vi "ESR Scanner - pulsed optimizer.vi"(0 "ESR Parameters":T1={"Window 1 time (s)"=0.012, "Window 2 time (s)"=5e-06, "Window 3 time (s) "=0.02, "Window 4 time (s)"=5e-07, "Window 4 channels"=[TRUE, FALSE, FALSE, TRUE], "Window 3 channels"=[TRUE, FALSE, TRUE, TRUE], "Window 2 channels"=[TRUE, FALSE, FALSE, TRUE], "Window 1 channels"=[TRUE, TRUE, FALSE, TRUE], "Path to ESR Burner"=path "C:/Users/Loncar/Desktop/ESR VIs - Srujan/Sam Kim/PB/ESRFreq.exe"}, 1 "MW start freq (GHz)":dbl=2.84, 2 "MW stop freq (GHz)":dbl=2.9, 3 "# freq points":i32=61, 4 "# scans before track":i32=50, 5 "#scan iterations":i32=50, 6 "IntGraph Refnum":refnum<vi>, 7 "Optimize Parameters":T2={"Volt Step"={"X"=0.01, "Y"=0.01, "Z"=0.0}, "Num Iterations"=1, "Dwell Time (ms)"=100, "Volts Range"={"X"=0.1, "Y"=0.1, "Z"=0.0}, "Method"={"X"=enum."Max", "Y"=enum."Max"}} {"Volts Range"."Z" min=0.0; "Volts Range"."Y" min=0.0; "Volts Range"."X" min=0.0; "Dwell Time (ms)" min=0; "Num Iterations" min=1 step=1; "Volt Step"."Z" min=0.0; "Volt Step"."Y" min=1e-06; "Volt Step"."X" min=1e-06}, 8 "XY Graph Refnum":refnum<vi>, 14 "Save avg spectrum data to spreadsheet?":bool, 15 "Path for avg spectrum spreadsheet":path=path "C:/experiment/data/may_15_2012/SIL1_NV1_pippin_uW_off", 16 "Save avg spectrum graph?":bool, 17 "Path for avg spectrum graph":path=path "C:/experiment/data/may_15_2012/SIL1_NV1_pippin_uW_off") -> ()   [LabVIEW 2012]
uses:
  Strict Type Def - Optimize Parameters Cluster.ctl
  ESR Window Parameters.ctl
  <vilib>/DAQmx/read.llb/DAQmx Read (Counter 1D U32 1Chan NSamp).vi
  Channels.vi
  <vilib>/DAQmx/miscellaneous.llb/DAQmx Fill In Error Info.vi
  Global Vars.vi
  <vilib>/Analysis/baseanly.llb/Mean (DBL).vi
  <vilib>/Utility/file.llb/Write To Spreadsheet File (DBL).vi
  <vilib>/Analysis/NI_AALBase.lvlib
panel:
  out "Counts vs. frequency":i32[][](graph)
  out "Avg ESR spectrum":cluster{"Y":dbl[], "Y":dbl[]}[](graph)
  # "Note:\nThis is not a standalone program. It is called from ScannerUI"
  # "Default PB connections:\nPB0 - MW switch\nPB1 - MW freq step\nPB2 - Counter sample clk\nPB3 - Green AOM"
  # "VI for ESR spectrum measurement\n08/26/2013, Srujan Meesala\n12/18/2013, Samuel Kim"
  # "Stop experiment and\nreset PulseBlaster"
  # "MW freq step\ndwell time"
  # "MW freq step"
  # "Wait"
  # "Fluorescence\ncounting"
  # "Ctr sample clk"
  # "Wait"
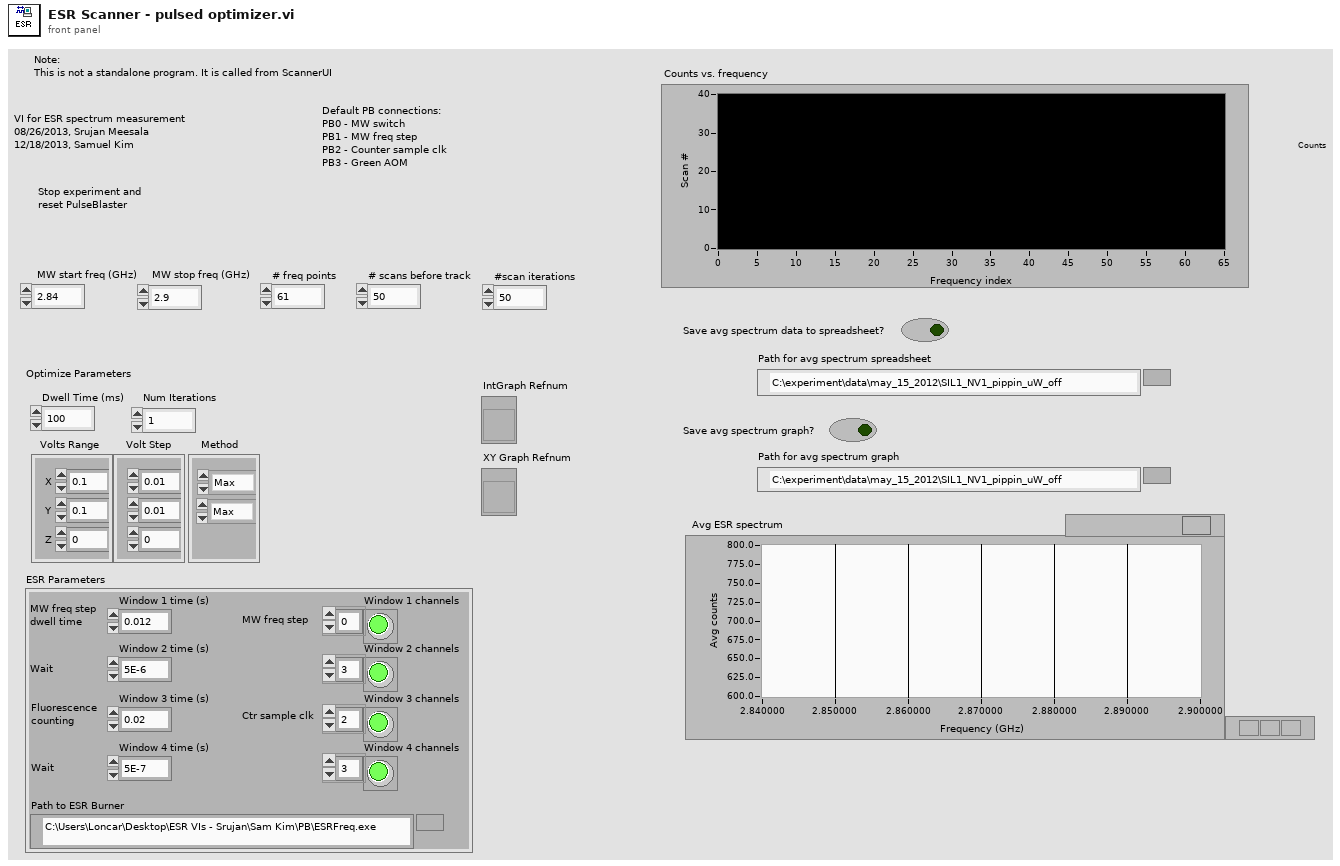
[diagram p1: front panel]
types:
  T1 = typedef "ESR Window Parameters.ctl" = cluster{"Window 1 time (s)":dbl, "Window 2 time (s)":dbl, "Window 3 time (s) ":dbl, "Window 4 time (s)":dbl, "Window 4 channels":bool[], "Window 3 channels":bool[], "Window 2 channels":bool[], "Window 1 channels":bool[], "Path to ESR Burner":path}
  T2 = typedef "Strict Type Def - Optimize Parameters Cluster.ctl" = cluster{"Volt Step":cluster{"X":dbl, "Y":dbl, "Z":dbl}, "Num Iterations":i32, "Dwell Time (ms)":i32, "Volts Range":cluster{"X":dbl, "Y":dbl, "Z":dbl}, "Method":cluster{"X":enum16{"Max", "Gaussian"}, "Y":enum16{"Max", "Gaussian"}}}
  T3 = typedef "imagedata.ctl" = cluster{"image type":i32, "image depth":i32, "image":u8[], "mask":u8[], "colors":u32[], "Rectangle":cluster{"left":i16, "top":i16, "right":i16, "bottom":i16}}
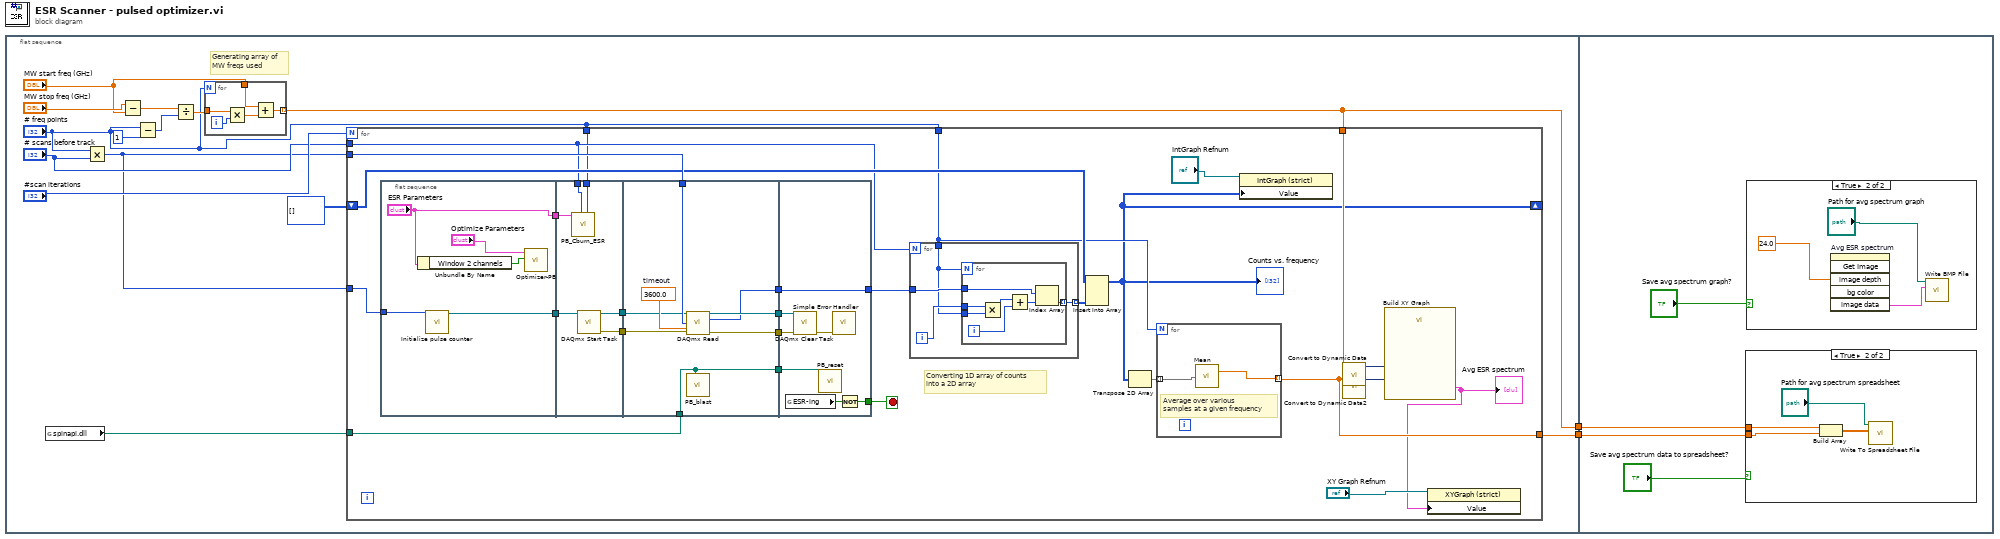
[diagram p0: block diagram]
diagram:
  n1 = flat-sequence {
    tunnel: [w8] -> w2
    tunnel: [w7] -> w1
    tunnel: w2 -> [w89]
    tunnel: w1 -> [w88]
    frame #0 {
      # "Generating array of\nMW freqs used"
      n2 = global read "Channels.vi" "spinapi.dll"() -> (w5:path)
      n3 = Multiply(x="# freq points", y="# scans before track") -> (x*y=w3:i32)
      n4 = Subtract(x="MW stop freq (GHz)", y="MW start freq (GHz)") -> (x-y=w14:dbl)
      n5 = Subtract(x="# freq points", y=u32 1 ("Reset Count")) -> (x-y=w15:u32)
      n6 = Divide(x=w14, y=w15) -> (x/y=w12:dbl)
      n7 = for {
        N: "# freq points" -> [_]
        tunnel: w12 -> [w86]
        tunnel: "MW start freq (GHz)" -> [w84]
        tunnel: [w83] -> w8 mode=indexing
        i -> [w87]
        n8 = Multiply(x=w86, y=w87) -> (x*y=w85:dbl)
        n9 = Add(x=w84, y=w85) -> (x+y=w83:dbl)
      }
      n10 = for {
        N: "#scan iterations" -> [_]
        tunnel: w5 -> [w18]
        tunnel: w3 -> [w43]
        tunnel: "# scans before track" -> [w24]
        tunnel: "# freq points" -> [w32]
        shift-right: [w28] -> _
        shift-left: i32[][] [] ("Flourescence Data") -> [w34]
        tunnel: w8 -> [w31]
        tunnel: [w30] -> w7
        tunnel: "# freq points" -> [w23]
        tunnel: w3 -> [w20]
        stop <- w17 stop-if-true
        # "Converting 1D array of counts \ninto a 2D array"
        n11 = flat-sequence {
          tunnel: ["ESR Parameters"] -> w25
          tunnel: w20 -> [w60]
          tunnel: [w59] -> w19
          tunnel: w25 -> [w62]
          tunnel: w24 -> [w64]
          tunnel: w23 -> [w63]
          tunnel: [w67] -> w22
          tunnel: [w66] -> w21
          tunnel: w19 -> [w65]
          tunnel: w43 -> [w74]
          tunnel: w18 -> [w71]
          tunnel: [w73] -> w42
          tunnel: [w72] -> w41
          tunnel: [w71] -> w40
          tunnel: [w68] -> w36
          tunnel: w22 -> [w70]
          tunnel: w21 -> [w69]
          tunnel: w42 -> [w79]
          tunnel: w41 -> [w80]
          tunnel: w40 -> [w82]
          tunnel: [w81] -> w35
          tunnel: w36 -> [w81]
          tunnel: [w76] -> w17
          frame #0 {
            n12 = Unbundle By Name("ESR Parameters") -> ("Window 2 channels"=w58:bool[])
            n13 = call "Initialize pulse counter.vi"("Samples per channel"=w60) -> ("DAQmx Task Name"=w59:refnum<k21>)  [unwired: 9 in, 1 out]
            n14 = call "Optimizer-PB.vi"("Optimize active channels"=w58, "Optimize Parameters"="Optimize Parameters") -> ()  [unwired: 9 in, 1 out]
          }
          frame #1 {
            n15 = call "PB_Cburn_ESR.vi"("# freq points"=w63, "# scans before track"=w64, "ESR Parameters"=w62) -> ()  [unwired: 9 in]
            n16 = call <vilib>:"DAQmx Start Task.vi"("task/channels in"=w65) -> ("task out"=w67:refnum<k21>, "error out"=w66:errorcluster)  [unwired: 13 in]
          }
          frame #2 {
            w75 = 3600.0  # timeout
            n17 = call-poly <vilib>:"DAQmx Read.vi"("task/channels in"=w70, "number of samples per channel"=w74, "timeout"=w75, "error in"=w69) -> ("task out"=w72:refnum<k21>, "data"=w68:u32[], "error out"=w73:errorcluster)  [unwired: 9 in]
            n18 = call "PB_blast.vi"("Path to spinapi.dll"=w71) -> ()  [unwired: 7 in]
          }
          frame #3 {
            n19 = global read "Global Vars.vi" "ESR-ing"() -> (w77:bool)
            n20 = call <vilib>:"DAQmx Clear Task.vi"("task in"=w80, "error in"=w79) -> ("error out"=w78:errorcluster)  [unwired: 13 in]
            n21 = call "PB_reset.vi"("Path to spinapi.dll"=w82) -> ()  [unwired: 7 in]
            n22 = call <vilib>:"Simple Error Handler.vi"("error in (no error)"=w78) -> ()  [unwired: 4 in, 5 out]
            n23 = Not(x=w77) -> (.not. x?=w76:bool)
          }
        }
        n24 = for {
          N: w24 -> [_]
          tunnel: w35 -> [w47]
          tunnel: w32 -> [w44]
          tunnel: [w46] -> w33 mode=indexing
          i -> [w45]
          n25 = for {
            N: w44 -> [_]
            tunnel: w45 -> [w54]
            tunnel: w47 -> [w52]
            tunnel: [w51] -> w46 mode=indexing
            tunnel: w44 -> [w49]
            i -> [w50]
            n26 = Multiply(x=w54, y=w49) -> (x*y=w48:i32)
            n27 = Add(x=w48, y=w50) -> (x+y=w53:i32)
            n28 = Index Array(array=w52, index=w53) -> (element=w51:u32)
          }
        }
        n29 = Insert Into Array(array=w34, new element=w33) -> (w28:i32[][])  [unwired: 2 in]
        "Counts vs. frequency" <- w28
        n30 = Transpose 2D Array(2D array=w28) -> (transposed array=w37:i32[][])
        n31 = for {
          N: w32 -> [_]
          tunnel: [w56] -> w30 mode=indexing
          tunnel: w37 -> [w55] mode=indexing
          # "Average over various \nsamples at a given frequency"
          n32 = call-poly <vilib>:"Mean.vi"("X"=w55) -> ("mean"=w56:dbl)  [unwired: 1 out]
        }
        n33 = property class="IntGraph (strict)"(reference="IntGraph Refnum", "Value"=w28) -> ()  [unwired: 1 in, 2 out]
        n34 = call "Convert to Dynamic Data"("Array"=w31) -> ("Dynamic Data Type"=w39:dynamicdata)  [unwired: 3 in]
        n35 = call "Convert to Dynamic Data2"("Array"=w30) -> ("Dynamic Data Type"=w38:dynamicdata)  [unwired: 3 in]
        n36 = call "Build XY Graph"("Y Input"=w38, "X Input"=w39) -> ("XY Graph"=w26:cluster{"Y":dbl[], "Y":dbl[]}[])  [unwired: 3 in, 6 out]
        "Avg ESR spectrum" <- w26
        n37 = property class="XYGraph (strict)"(reference="XY Graph Refnum", "Value"=w26) -> ()  [unwired: 1 in, 2 out]
      }
    }
    frame #1 {
      n38 = case shown="True" "Save avg spectrum data to spreadsheet?" {
        tunnel: w89 -> [_ w93]
        tunnel: w88 -> [_ w92]
        frame False {
        }
        frame True {
          n39 = Build Array(w93, w92) -> (w94:dbl[][])
          n40 = call-poly <vilib>:"Write To Spreadsheet File.vi"("2D data"=w94, "file path (dialog if empty)"="Path for avg spectrum spreadsheet") -> ()  [unwired: 6 in, 1 out]
        }
      }
      n41 = case shown="True" "Save avg spectrum graph?" {
        frame False {
        }
        frame True {
          n42 = invoke on="Avg ESR spectrum" class="XYGraph (strict)" method="Get Image"("image depth"=24.0 ("Initial Delay")) -> ("image data"=w96:T3)  [unwired: 5 in, 5 out]
          n43 = call <vilib>:"Write BMP File.vi"("image data"=w96, "path to BMP file"="Path for avg spectrum graph") -> ()  [unwired: 8 in, 2 out]
        }
      }
    }
  }
